vi "Do.vi"(8 "error in (no error)":errorcluster, 10 "Actor in":refnum<class "Actor.lvclass">, 11 "Update RD Write MSG":refnum<class "Update RD Write MSG.lvclass">) -> (0 "error out":errorcluster, 2 "Actor out":refnum<class "Actor.lvclass">)   [LabVIEW 2014, in "Instrument Library.lvlib" / "Update RD Write MSG.lvclass"]
doc: "(<B>Filename</B>: Actor Framework.lvlib:Message.lvclass:Do.vi)\n\nDefines what a message does when it is received by an actor. Generally, a message instructs an actor to invoke one of its methods. By default, this method does nothing. A child class must override it to define behavior. Create a child class by using the Actor Framework Message Maker dialog box."
uses:
  Update RD Write MSG.lvclass
  Instr Actor.lvclass
  CRDS/Commands/Write Ringdowns/Set Write Ringdowns CMD.lvclass
  <vilib>/ActorFramework/Actor/Actor.lvclass
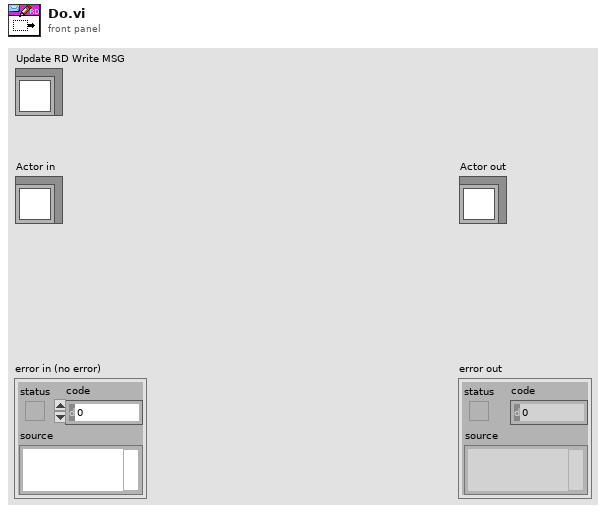
[diagram p1: front panel]
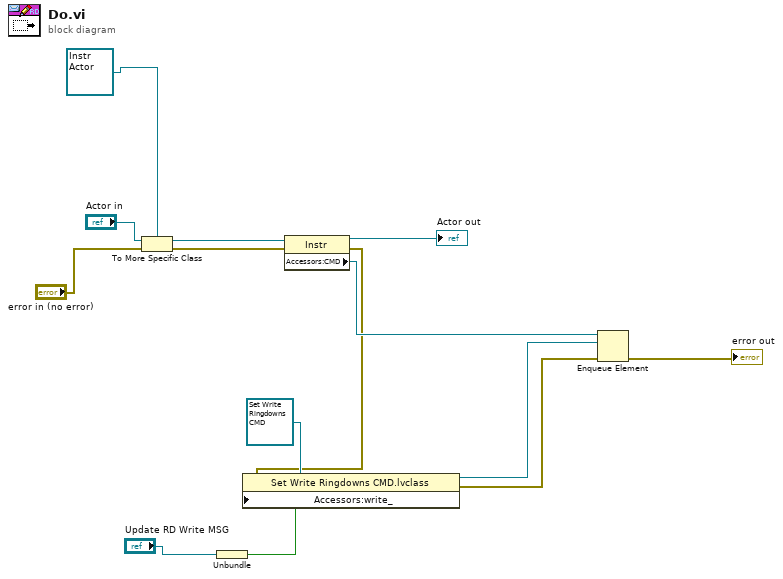
[diagram p0: block diagram]
diagram:
  n1 = To More Specific Class(target class=refnum<class "Instr Actor.lvclass"> refnum ("Instrument Lib:Instr"), reference="Actor in", error in="error in (no error)") -> (specific class reference=w12:refnum<class "Instr Actor.lvclass">, error out=w4:errorcluster)
  n2 = Unbundle("Update RD Write MSG") -> (w9:bool)
  n3 = property class="Instr"(reference=w12, error in=w4) -> (reference out=→"Actor out":refnum<class "Instr Actor.lvclass">, error out=w3:errorcluster, "Accessors:CMD"=w8:refnum<queue>)
  n4 = property class="Set Write Ringdowns CMD.lvclass"(reference=refnum<class "Set Write Ringdowns CMD.lvclass"> refnum ("Set Write Ringdowns CMD"), error in=w3, "Accessors:write_"=w9) -> (reference out=w7:refnum<class "Set Write Ringdowns CMD.lvclass">, error out=w2:errorcluster)
  n5 = Enqueue Element(queue=w8, element=w7, error in (no error)=w2) -> (error out=→"error out":errorcluster)  [unwired: 1 in, 2 out]
